vi "getiduserbyname.vi"(1 "name":string, 2 "Fichier DB":string) -> (0 "id":dbl)   [LabVIEW 2024]
uses:
  <vilib>/drjdpowell/SQLite Library/SQL Connection/Open (string).vi
  <vilib>/drjdpowell/SQLite Library/SQL Connection/Execute SQL.vi
  <vilib>/drjdpowell/SQLite Library/SQL Connection/Connection.lvclass
  <vilib>/drjdpowell/SQLite Library/SQLite.lvlib
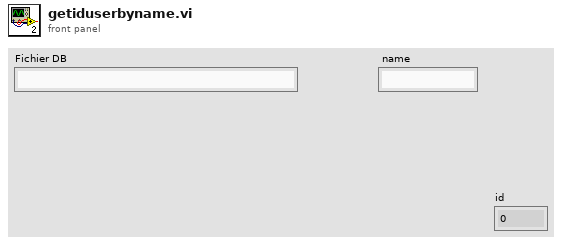
[diagram p1: front panel]
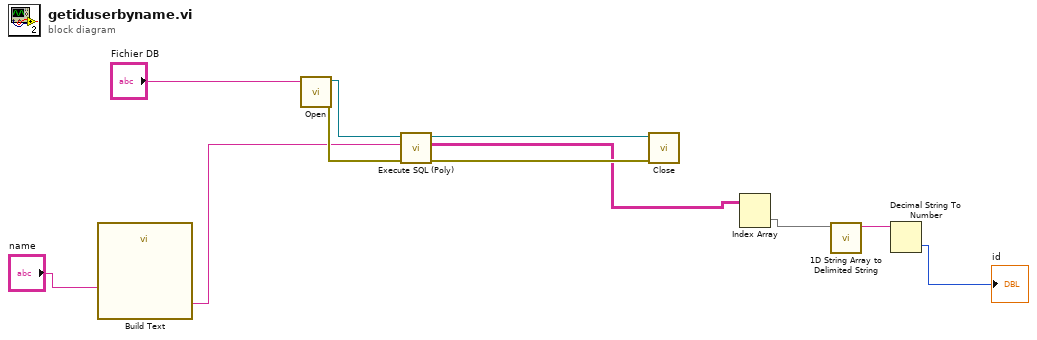
[diagram p0: block diagram]
diagram:
  n1 = call "Build Text"("name"="name") -> ("Result"=w6:string)  [unwired: 13 in, 1 out]
  n2 = call-poly <vilib>:"Open.vi"("db file"="Fichier DB") -> ("error out"=w8:errorcluster, "SQLite Connection"=w9:refnum<class "Connection.lvclass">)  [unwired: 9 in]
  n3 = call-poly <vilib>:"Execute SQL (Poly).vi"("error in (no error)"=w8, "SQL"=w6, "SQLite Connection in"=w9) -> ("error out"=w10:errorcluster, "Result Set"=w4:string[][], "SQLite Connection"=w11:refnum<class "Connection.lvclass">)  [unwired: 5 in, 1 out]
  n4 = call-dynamic "Close.vi"("error in (no error)"=w10, "SQLite Connection in"=w11) -> ()  [unwired: 9 in, 1 out]
  n5 = Index Array(array=w4) -> (element=w5:string[])  [unwired: 2 in]
  n6 = call <vilib>:"1D String Array to Delimited String.vi"("string array"=w5) -> ("delimited string"=w1:string)  [unwired: 10 in]
  n7 = Decimal String To Number(string=w1) -> (number=→"id":i32)  [unwired: 2 in, 1 out]
